vi "Execute.vi"(8 "Error In":errorcluster, 11 "Test Framework.lvclass":refnum<class "Test Framework.lvclass">) -> (0 "Error Out":errorcluster, 3 "Test Framework.lvclass Out":refnum<class "Test Framework.lvclass">)   [LabVIEW 2020, in "Test Framework.lvclass"]
uses:
  Test Framework.lvclass
  Controls/Control references.ctl
  Support VIs/Message Queue/States.ctl
  Controls/Display states.ctl
  Test Framework.lvclass/Test Framework.ctl
  XML Handler/XML Handler.lvclass/XML Handler.ctl
  Instruments/Vector Network Analyzer/Vector Network Analyzer.lvclass
  Path Control/PathControl.lvclass/PathControl.ctl
  Controls/Temperature and voltage modes.ctl
  <vilib>/sound2/lvsound2.llb/Sampling Mode.ctl
  Support VIs/Message Queue/Enqueue Message (Single).vi
  Support VIs/Message Queue/Enqueue Message (Array).vi
  <vilib>/sound2/lvsound2.llb/Sound File Info (path).vi
  <vilib>/sound2/lvsound2.llb/Sound Output Write (DBL).vi
  Devices/Toggle 8/WS1021/WS1021 GUI.vi
  <vilib>/Utility/xml.llb/Write to XML File(string).vi
  Devices/Device.lvclass
  Support VIs/User Event - Stop/User Event - Stop.lvlib
  Support VIs/Message Queue/Message Queue.lvlib
  Path Control/PathControl.lvclass
  XML Handler/XML Handler.lvclass
  Devices/Toggle 8/WS1021/WS1021.lvclass
panel:
  out "Time String":string
  in  "OpenFolder":bool
  in  "Device Information":string[][](array[string])
  in  "File Name":string
  out "Progress Bar":u8(slide) scale=0.0..100.0
  in  "Data Path":path
  in  "Exit Button":bool
  in  "Run Measurements Button":bool
  in  "Configure Measurements Button":bool
  in  "Calibrate Paths Button":bool
  in  "Conf Device Button":bool
  in  "Conf temp and DC Button":bool
  in  "Assign Instr Button":bool
  in  "Test Listbox":i32(listbox) caption="Measurement"
  # "%"
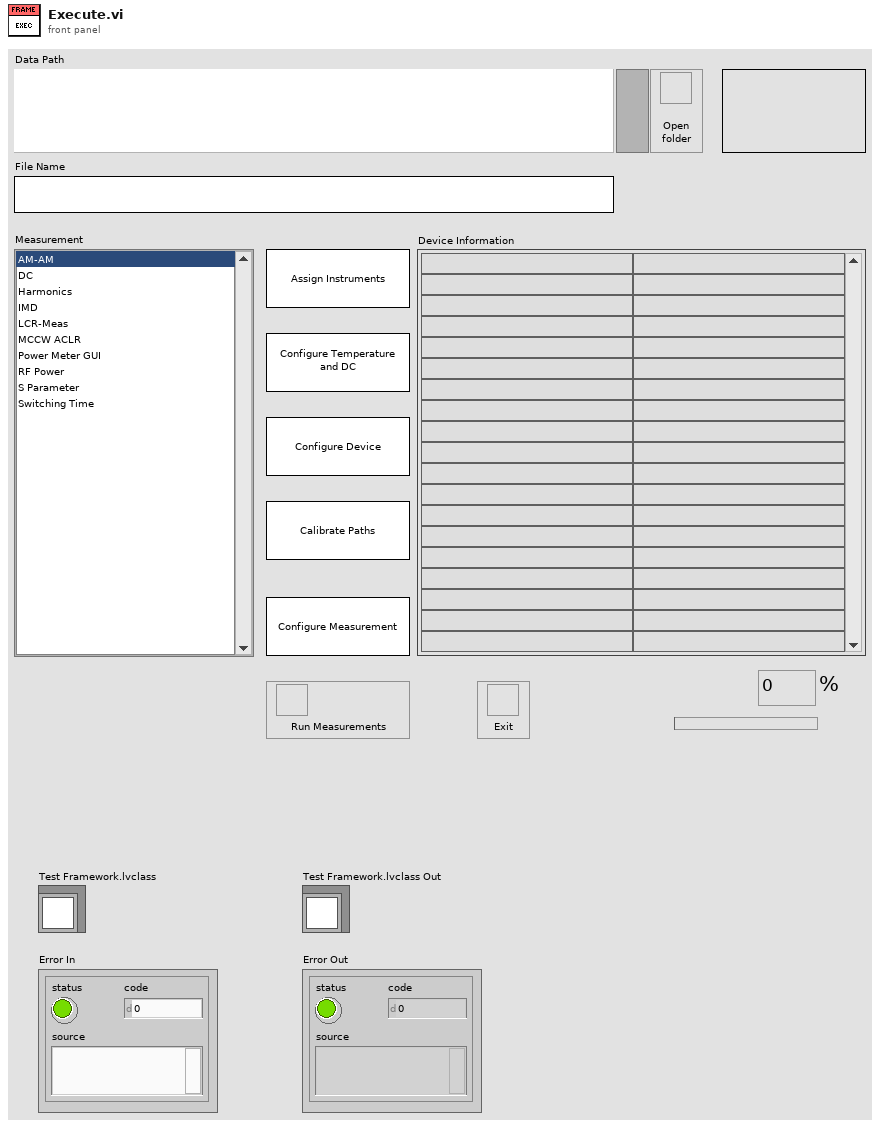
[diagram p1: front panel]
types:
  T1 = enum32{"invalid app kind", "Development System", "Run Time System", "Student Edition", "Embedded LabVIEW", "Evaluation", "Custom"}
  T2 = typedef "Test Framework.lvclass/Control references.ctl" = cluster{"Assign Instr Button Ref":refnum<vi>, "Conf temp/voltage Button Ref":refnum<vi>, "Conf Device Button Ref":refnum<vi>, "Calibrate Path Button Ref":refnum<vi>, "Configure Meas Button Ref":refnum<vi>, "Run Measurements Button Ref":refnum<vi>, "Exit Button Ref":refnum<vi>, "Test Listbox Ref":refnum<vi>, "Data Path Ref":refnum<vi>, "File Name":refnum<vi>, "CtrlWithKeyFocus":refnum<vi>}
  T3 = typedef "Message Queue.lvlib/All Message Queues.ctl" = cluster{"UI":refnum<queue>}
  T4 = enum16{"open", "replace", "create", "open or create", "replace or create", "replace or create with confirmation"}
  T5 = typedef "Test Framework.lvclass/Display states.ctl" = enum16{"Start up", "Measurements Running"}
  T6 = typedef "Message Queue.lvlib/States.ctl" = enum16{"Init", "Update Display", "Assign Instruments", "Configure Evironmental", "Configure Device", "Update device info", "Calibrate Path", "Configure Test", "Init XML", "Init Environmental", "Next Environmental", "Run Tests", "Cancel Tests", "Change Data Path", "Update test list", "Finish test", "Exit", "Error", "Menu Selection"}
  T7 = typedef "Test Framework.lvclass/Temperature and voltage modes.ctl" = cluster{"Temperature mode":enum16{"Automatic", "Manual", "Off"}, "DC-Power mode":enum16{"Automatic", "Manual", "Off"}, "PSU sweep mode":bool, "Turn off after measurement":bool}
  T8 = enum32{"Invalid", "Standard", "Closed", "Hidden", "Minimized", "Maximized"}
  T9 = typedef "Device.lvclass/Device Information Cluster.ctl" = cluster{"Device Info":string[][], "Default Values":T10[], "Fetched info":string[][]}
  T10 = typedef "PIC-Device.lvclass/Register to Write.ctl" = cluster{"Register":u32, "Value":u32, "Dev Address":u32, "Physical Adress":u32}
  T11 = cluster{"Instrument Name":string, "Instrument.lvclass":refnum<class "Instrument.lvclass">, "Reference":bool}[]
  T12 = cluster{"Restart?":bool, "User system setting file":path}
  T13 = typedef "Test Framework.lvclass/Temperature and voltage array.ctl" = cluster{"Temperature [C]":dbl, "Soak time [m]":dbl, "PSUs":cluster{"Enabled":bool, "Source":enum32{"Voltage", "Current"}, "Drive (V/A)":dbl, "Sweep (V/A)":string, "Limit (A/V)":dbl, "PSU alias":string, "PSU info":cluster{"ID":string, "Address":string, "Channel":u8}}[]}[]
  T14 = cluster{"Temperature control array":T13, "Temperature mode":T7}
  T15 = typedef "Sampling Mode.ctl" = i32
  T16 = typedef "Sound Data Format.ctl" = cluster{"sample rate (S/s)":dbl, "number of channels":i32, "bits per sample":i32}
  T17 = typedef "Sound Output Task ID.ctl" = u32
  T18 = enum32{"Bad", "Idle", "Run top level", "Running"}
  T19 = typedef "LVPoint32TypeDef.ctl" = cluster{"Horizontal":i32, "Vertical":i32}
  T20 = cluster{"appended path":path, "appended path":path}
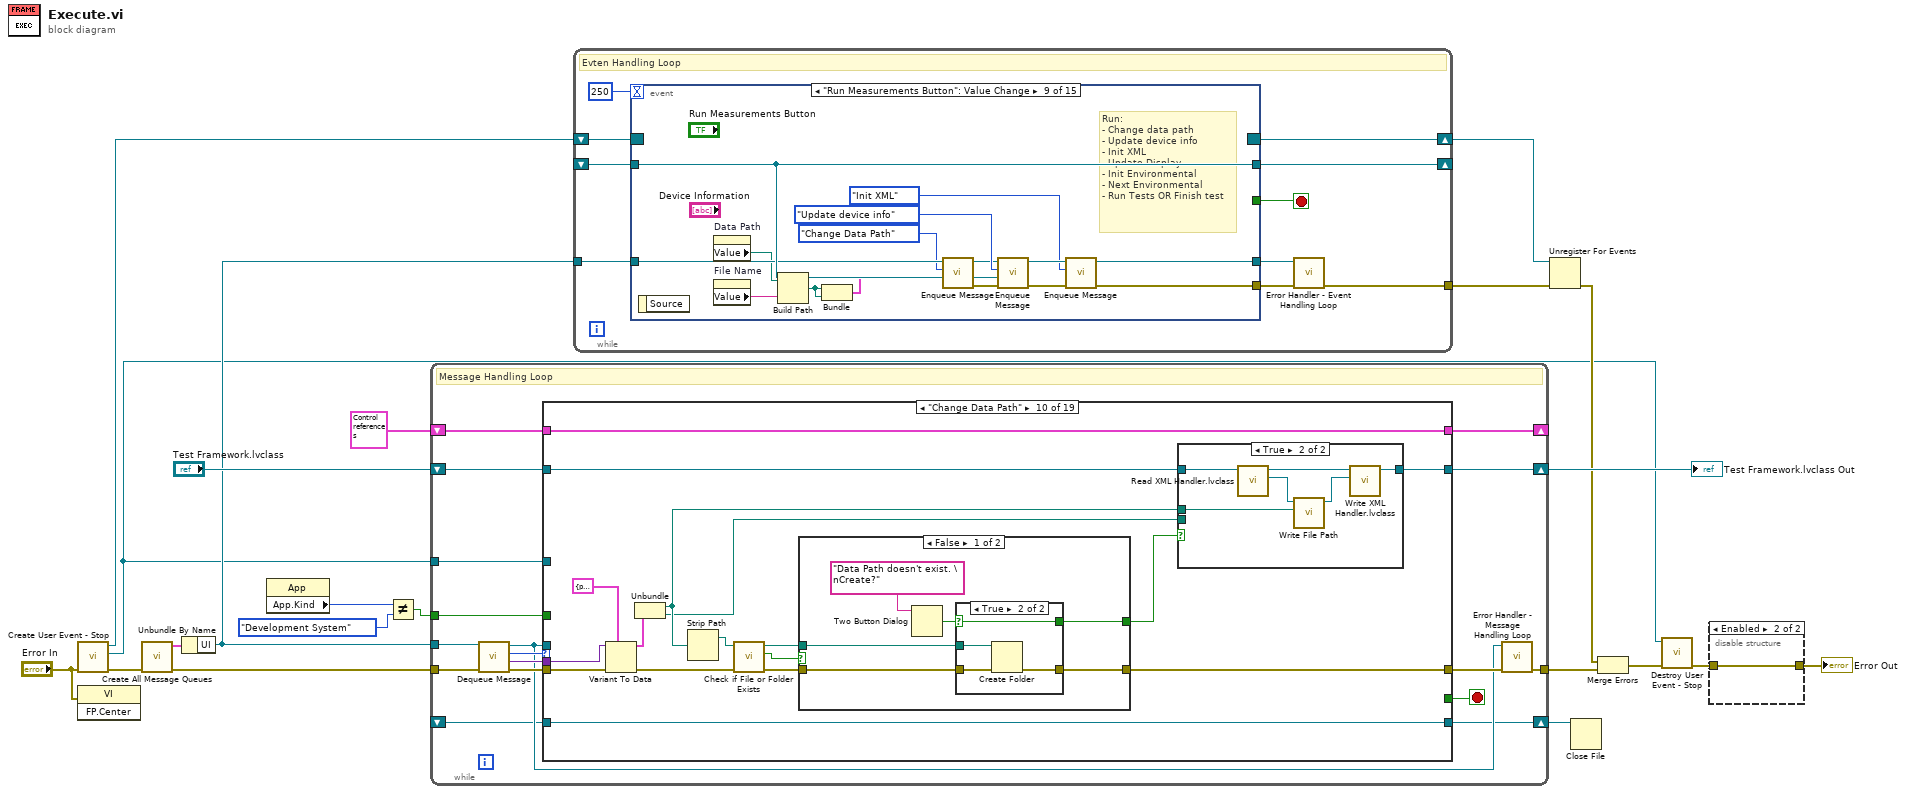
[diagram p0: block diagram]
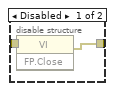
[diagram p2: hidden frame]
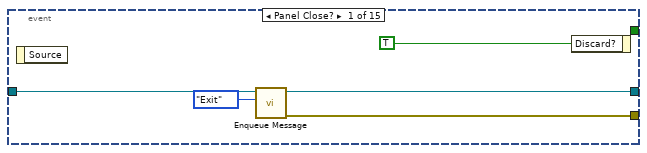
[diagram p3: hidden frame]
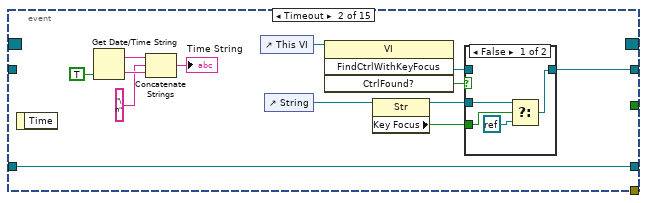
[diagram p4: hidden frame]
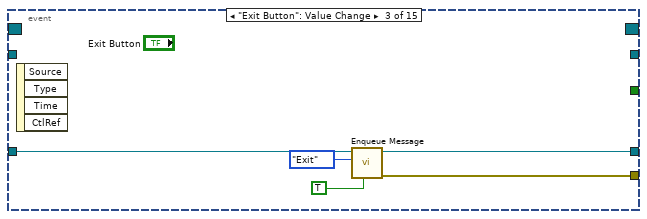
[diagram p6: hidden frame]
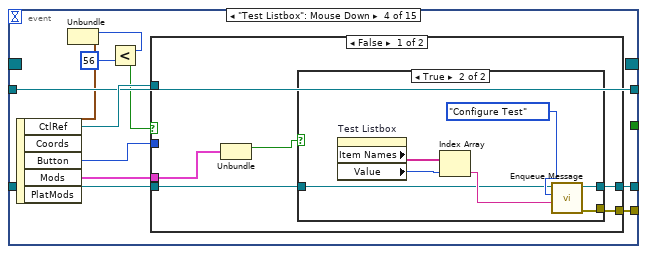
[diagram p7: hidden frame]
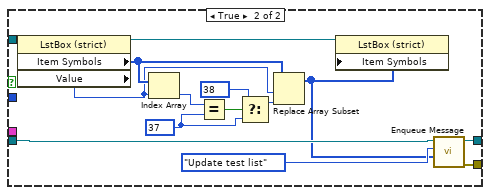
[diagram p9: hidden frame]
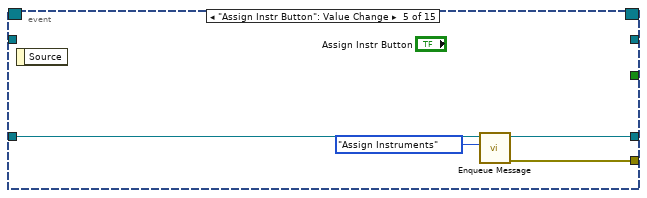
[diagram p10: hidden frame]
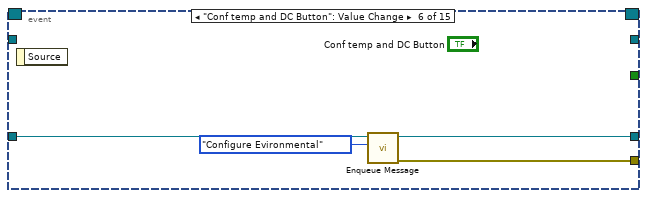
[diagram p11: hidden frame]
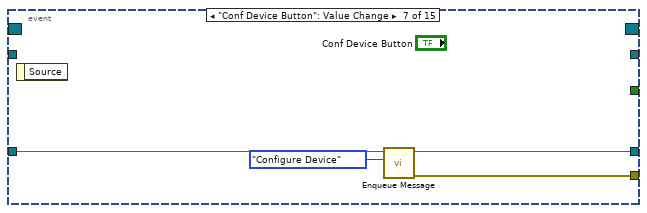
[diagram p12: hidden frame]
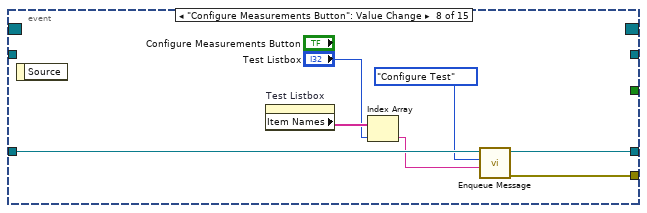
[diagram p13: hidden frame]
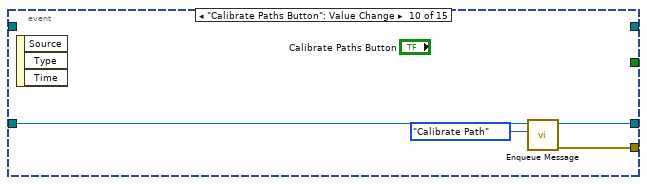
[diagram p14: hidden frame]
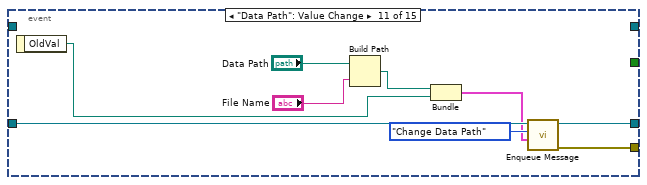
[diagram p15: hidden frame]
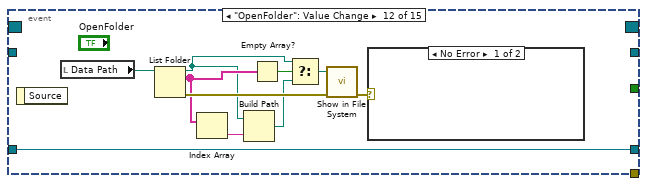
[diagram p16: hidden frame]
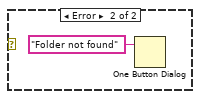
[diagram p17: hidden frame]
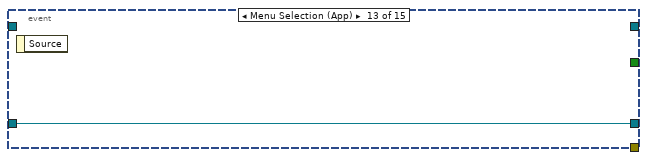
[diagram p18: hidden frame]
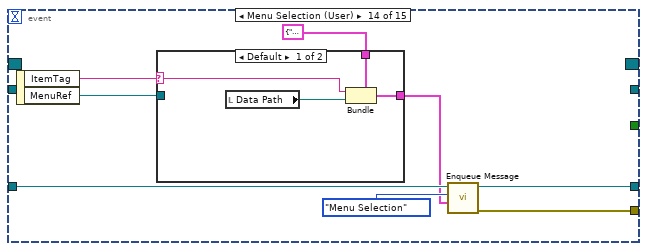
[diagram p19: hidden frame]
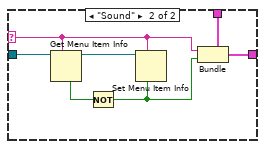
[diagram p20: hidden frame]
diagram:
  n1 = call "Create User Event - Stop.vi"("error in (no error)"="Error In") -> ("error out"=w21:errorcluster, "User Event - Stop"=w10:refnum<user-event>, "Stop Event Registration Refnum"=w15:refnum<event-registration>)  [unwired: 8 in]
  n2 = invoke class="VI" method="FP.Center"(error in="Error In") -> ()  [unwired: 2 in, 3 out]
  n3 = call "Create All Message Queues.vi"("error in (no error)"=w21) -> ("error out"=w20:errorcluster, "Message Queues out"=w19:T3)  [unwired: 9 in]
  n4 = Unbundle By Name(w19) -> ("UI"=w16:refnum<queue>)
  n5 = property class="App"() -> ("App.Kind"=w2:T1)  [unwired: 2 in, 2 out]
  n6 = Not Equal?(x=w2, y=T1."Development System" ("Application:Kind")) -> (x != y?=w1:bool)
  n7 = while {
    tunnel: w16 -> [w37]
    shift-right: [w32] -> w17
    shift-left: "Test Framework.lvclass" -> [w33]
    tunnel: w20 -> [w38]
    tunnel: w10 -> [w31]
    tunnel: [w27] -> w11
    shift-right: [w25] -> _
    shift-left: T2 {"Assign Instr Button Ref"=refnum, "Conf temp/voltage Button Ref"=refnum, "Conf Device Button Ref"=refnum, "Calibrate Path Button Ref"=refnum, "Configure Meas Button Ref"=refnum, "Run Measurements Button Ref"=refnum, "Exit Button Ref"=refnum, "Test Listbox Ref"=refnum, "Data Path Ref"=refnum, "File Name"=refnum, "CtrlWithKeyFocus"=refnum} ("Cluster") -> [w26]
    shift-right: [w23] -> w4
    shift-left: _ -> [w24]
    tunnel: w1 -> [w22]
    stop <- w30 stop-if-true
    # "Message Handling Loop"
    n8 = call "Dequeue Message.vi"("error in (no error)"=w38, "Message Queue"=w37) -> ("error out"=w35:errorcluster, "Message Data"=w34:variant, "Message"=w36:T6, "dup Message Queue"=w28:refnum<queue>)  [unwired: 6 in]
    n9 = case shown="\"Change Data Path\"" w36 {
      tunnel: w28 -> [w66 _ _ _ _ _ _ w213 _ _ w287 w297 _ w326 w363 _ w410 w434 _]
      tunnel: w35 -> [w45 w91 w99 w106 w140 w161 w192 w220 w239 w256 w292 w305 w315 w331 w365 w391 w414 w419 w470]
      tunnel: w34 -> [_ w88 _ _ w139 _ w191 _ _ w255 _ w304 _ w324 _ w389 _ _ w469]
      tunnel: w33 -> [w84 w93 w97 w107 w149 w167 w195 w211 w238 w254 w283 w306 w314 w330 w361 w395 w413 w417 w461]
      tunnel: [w47 w93 w96 w102 w150 w168 w194 w222 w238 w253 w284 w306 w310 w329 w364 w386 w412 w421 w460] -> w32
      tunnel: [w67 w92 w98 w105 w141 w171 w193 w215 w239 w240 w288 w295 w311 w325 w362 w390 w409 w428 w466] -> w29
      tunnel: w31 -> [_ _ _ _ _ _ _ _ _ _ w291 _ _ _ _ _ _ _ w458]
      tunnel: [_ _ _ _ _ _ _ _ _ _ TRUE _ _ _ _ _ _ _ w457] -> w30
      tunnel: w26 -> [w78 w85 w95 w108 w136 w160 w187 w221 w237 w252 w286 w300 w309 w328 w366 w396 w415 w423 w471]
      tunnel: [w77 w85 w95 w108 w135 w160 w187 w221 w237 w252 w286 w300 w309 w328 w366 w396 w415 w423 w471] -> w25
      tunnel: w24 -> [_ w86 w94 w100 w142 w159 w186 w201 w236 w251 w285 w294 w307 w322 w341 w385 w401 w426 w468]
      tunnel: [w53 w86 w94 w100 w142 w159 w186 w201 w236 w251 w285 w293 w307 w322 w341 w385 w401 w426 w468] -> w23
      tunnel: w22 -> [_ _ _ _ _ _ _ _ _ _ _ _ _ _ _ _ _ _ w459]
      frame "Init" {
        n10 = call "Read Test Listbox.vi"("Test Framework in"=w84) -> ("Value"=w81:i32, "Symbols"=w82:i32[], "Measurement Names"=w83:string[], "Test Framework out"=w80:refnum<class "Test Framework.lvclass">)  [unwired: 7 in]
        n11 = call "Get AppData Directory.vi"("Error In"=w45) -> ("Error Out"=w44:errorcluster, "Folder path"=w43:path)  [unwired: 8 in, 1 out]
        n12 = property on="Test Listbox" class="LstBox (strict)"("Item Names"=w83, "Item Symbols"=w82, "Value"=w81) -> ()  [unwired: 2 in, 2 out]
        n13 = call "Read XML Handler.lvclass.vi"("Test Framework in"=w80) -> ("XML Handler.lvclass"=w79:refnum<class "XML Handler.lvclass">, "Test Framework out"=w60:refnum<class "Test Framework.lvclass">)  [unwired: 9 in]
        n14 = call "Read File Path.vi"("XML Handler in"=w79) -> ("File Path"=w62:path)  [unwired: 9 in, 1 out]
        n15 = call-dynamic "Read Current Device.vi"("Test Framework in"=w60) -> ("Current Device.lvclass"=w61:refnum<class "Device.lvclass">, "Test Framework out"=w48:refnum<class "Test Framework.lvclass">)  [unwired: 9 in]
        n16 = Strip Path(path=w62) -> (stripped path=w63:path)  [unwired: 1 out]
        n17 = call <vilib>:"Get File Extension.vi"("file"=w62) -> ("filename without extension"=w41:string)  [unwired: 6 in, 4 out]
        n18 = Build Path(base path=w43, name or relative path="Error Log.txt") -> (appended path=w56:path)
        n19 = call-dynamic "Read Device Information.vi"("Device in"=w61) -> ("Device Info"=w59:T9[])  [unwired: 8 in, 2 out]
        n20 = Empty String/Path?(string/path=w41) -> (empty?=w42:bool)
        n21 = property on="Data Path" class="Path"("Value"=w63) -> ()  [unwired: 2 in, 2 out]
        n22 = Open/Create/Replace File(file path (use dialog)=w56, error in=w44, operation (0:open)=T4."open or create") -> (refnum out=w53:refnum<file>, error out=w52:errorcluster)  [unwired: 3 in, 1 out]
        n23 = Select(t="results", s=w42, f=w41) -> (s? t:f=w39:string)
        n24 = Index Array(array=w59) -> (element=w58:T9)  [unwired: 1 in]
        n25 = call-dynamic "Read Play sound when done.vi"("Test Framework in"=w48) -> ("Play sound when done"=w46:bool, "Test Framework out"=w47:refnum<class "Test Framework.lvclass">)  [unwired: 9 in]
        n26 = property on="File Name" class="Str"("Value"=w39) -> ()  [unwired: 2 in, 2 out]
        n27 = Unbundle By Name(w58) -> ("Device Info"=w57:string[][])
        n28 = control-ref of="Assign Instr Button"() -> (w76:refnum<vi>)
        n29 = control-ref of="Conf temp and DC Button"() -> (w75:refnum<vi>)
        n30 = control-ref of="Conf Device Button"() -> (w74:refnum<vi>)
        n31 = control-ref of="Calibrate Paths Button"() -> (w73:refnum<vi>)
        n32 = control-ref of="Configure Measurements Button"() -> (w72:refnum<vi>)
        n33 = control-ref of="Run Measurements Button"() -> (w71:refnum<vi>)
        n34 = control-ref of="Exit Button"() -> (w70:refnum<vi>)
        n35 = control-ref of="Test Listbox"() -> (w69:refnum<vi>)
        n36 = control-ref of="File Name"() -> (w51:refnum<vi>)
        n37 = control-ref of="Data Path"() -> (w68:refnum<vi>)
        n38 = local write "Device Information"(w57) -> ()
        n39 = Current VI's Menubar() -> (w50:refnum<k9>)
        n40 = Set Menu Item Info(6:w46, 7:"Sound" ("item tag"), 11:w50) -> ()  [unwired: 4 in, 2 out]
        n41 = Bundle By Name(cluster=w78, "Assign Instr Button Ref"=w76, "Conf temp/voltage Button Ref"=w75, "Conf Device Button Ref"=w74, "Calibrate Path Button Ref"=w73, "Configure Meas Button Ref"=w72, "Run Measurements Button Ref"=w71, "Exit Button Ref"=w70, "Test Listbox Ref"=w69, "Data Path Ref"=w68, "File Name"=w51) -> (w77:T2)
        n42 = call-poly "Enqueue Message.vi"("error in (no error)"=w52, "Message Data"=Display_states."Start up" ("type"), "Message"=States."Update Display", "Message Queue"=w66) -> ("error out"=w67:errorcluster)  [unwired: 6 in, 1 out]
      }
      frame "Update Display" {
        n43 = Variant To Data(error in=w91, type=Display_states."Start up", Variant=w88) -> (data=w90:T5, error out=w89:errorcluster)
        n44 = call "Update display.vi"("Error In"=w89, "Display states"=w90, "Cluster"=w85) -> ("Error Out"=w92:errorcluster)  [unwired: 8 in]
      }
      frame "Configure Evironmental" {
        n45 = call "Configure Environment.vi"("error in (no error)"=w99, "Test Framework in"=w97) -> ("error out"=w98:errorcluster, "Test Framework out"=w96:refnum<class "Test Framework.lvclass">)  [unwired: 8 in]
      }
      frame "Configure Device" {
        n46 = local read "Device Information"() -> (w101:string[][])
        n47 = call "Select Device.vi"("Error In"=w106, "Test Framework.lvclass"=w107) -> ("Error Out"=w105:errorcluster, "Test Framework out"=w103:refnum<class "Test Framework.lvclass">)  [unwired: 8 in]
        n48 = call-dynamic "Read Current Device.vi"("Test Framework in"=w103) -> ("Current Device.lvclass"=w104:refnum<class "Device.lvclass">, "Test Framework out"=w102:refnum<class "Test Framework.lvclass">)  [unwired: 9 in]
        n49 = disable-structure shown="Disabled" {
          disable-tunnel: w104 -> [w114 _]
          disable-tunnel: w101 -> [w112 _]
          frame Disabled {
            n50 = call-dynamic "Read Device Information.vi"("Device in"=w114) -> ("Device Info"=w113:T9[])  [unwired: 8 in, 2 out]
            n51 = for {
              tunnel: w113 -> [w121] mode=indexing
              tunnel: [w117] -> w110 mode=indexing if=w116
              shift-right: [w115] -> w111
              shift-left: w112 -> [w120]
              n52 = Index Array(array=w120) -> (element #1=w119:string[], element #2=w118:string[])  [unwired: 4 in]
              n53 = for {
                tunnel: w119 -> [w132] mode=indexing
                tunnel: w118 -> [w126] mode=indexing
                tunnel: [w131] -> w115 mode=indexing
                tunnel: [w122] -> w116
                tunnel: w121 -> [w128]
                tunnel: [w123] -> w117
                stop <- w122 continue-if-true
                n54 = Unbundle By Name(w128) -> ("Fetched info"=w130:string[][])
                n55 = Index Array(array=w130) -> (element=w129:string[])  [unwired: 2 in]
                n56 = Unbundle(w129) -> (w125, w124)
                n57 = Not Equal?(x=w132, y=w125) -> (x != y?=w122:bool)
                n58 = Select(t=w126, s=w122, f=w124) -> (s? t:f=w127:string)
                n59 = Build Array(w132, w127) -> (w131:string[])
                n60 = Build Array(w125, w124) -> (w123:void[])
              }
            }
            n61 = Insert Into Array(array=w111, new element=w110) -> (w109:string[][])  [unwired: 2 in]
            n62 = local write "Device Information"(w109) -> ()
          }
          frame Enabled {
          }
        }
      }
      frame "Update device info" {
        n63 = Variant To Data(error in=w140, type=refnum<vi> refnum ("CtrlWithKeyFocus"), Variant=w139) -> (data=w137:refnum<vi>, error out=w141:errorcluster)
        n64 = call-dynamic "Read Current Device.vi"("Test Framework in"=w149) -> ("Current Device.lvclass"=w145:refnum<class "Device.lvclass">, "Test Framework out"=w144:refnum<class "Test Framework.lvclass">)  [unwired: 9 in]
        n65 = Bundle By Name(cluster=w136, "CtrlWithKeyFocus"=w137) -> (w135:T2)
        n66 = local read "Device Information"() -> (w134:string[][])
        n67 = for {
          tunnel: w134 -> [w153] mode=indexing
          tunnel: [w153] -> w133 mode=indexing if=w151
          n68 = Index Array(array=w153, index=1) -> (element=w154:string)
          n69 = Empty String/Path?(string/path=w154) -> (empty?=w152:bool)
          n70 = Not(x=w152) -> (.not. x?=w151:bool)
        }
        n71 = call-dynamic "Read Device Information.vi"("Device in"=w145) -> ("Device Info"=w148:T9[], "Device out"=w146:refnum<class "Device.lvclass">)  [unwired: 8 in, 1 out]
        n72 = for {
          tunnel: w148 -> [w158] mode=indexing
          tunnel: [w157] -> w147 mode=indexing
          tunnel: w133 -> [w156]
          n73 = Bundle By Name(cluster=w158, "Device Info"=w156) -> (w157:T9)
        }
        n74 = call-dynamic "Write Device Information.vi"("Device Info"=w147, "Device in"=w146) -> ("Device out"=w143:refnum<class "Device.lvclass">)  [unwired: 8 in, 1 out]
        n75 = call-dynamic "Write Current Device.vi"("Current Device.lvclass"=w143, "Test Framework in"=w144) -> ("Test Framework out"=w150:refnum<class "Test Framework.lvclass">)  [unwired: 9 in]
      }
      frame "Calibrate Path" {
        n76 = call "Read PathControl.lvclass.vi"("Test Framework in"=w167) -> ("PathControl.lvclass"=w163:refnum<class "PathControl.lvclass">, "Test Framework out"=w170:refnum<class "Test Framework.lvclass">)  [unwired: 9 in]
        n77 = call "Read Instrumentes to Use.vi"("Test Framework in"=w167) -> ("Instrumentes to Use"=w166:T11)  [unwired: 9 in, 1 out]
        n78 = call "Find Instrument.vi"("Instrument Name"="Vector Network Analyzer", "Instrumentes to Use"=w166) -> ("Instrument Found?"=w164:bool, "Instrument.lvclass"=w162:refnum<class "Instrument.lvclass">)  [unwired: 8 in]
        n79 = case shown="True" w164 {
          tunnel: [w180 w185] -> w171
          tunnel: [w179 w184] -> w169
          tunnel: w163 -> [w177 w181]
          tunnel: w162 -> [w176 _]
          tunnel: w161 -> [w173 w183]
          frame True {
            n80 = To More Specific Class(target class=refnum<class "Vector Network Analyzer.lvclass"> refnum ("Vector Network Analyzer.lvclass"), reference=w176) -> (specific class reference=w174:refnum<class "Vector Network Analyzer.lvclass">)  [unwired: 1 in, 1 out]
            n81 = call "Write Vector Network Analyzer.lvclass.vi"("Vector Network Analyzer.lvclass"=w174, "PathControl in"=w177) -> ("PathControl out"=w178:refnum<class "PathControl.lvclass">)  [unwired: 9 in]
            n82 = call "Calibrate Path User Interface.vi"("error in (no error)"=w173, "VNA present"=TRUE ("VNA pressent"), "PathControl in"=w178) -> ("error out"=w180:errorcluster, "PathControl out"=w179:refnum<class "PathControl.lvclass">)  [unwired: 7 in]
          }
          frame False {
            n83 = call "Calibrate Path User Interface.vi"("error in (no error)"=w183, "VNA present"=FALSE ("VNA pressent"), "PathControl in"=w181) -> ("error out"=w185:errorcluster, "PathControl out"=w184:refnum<class "PathControl.lvclass">)  [unwired: 7 in]
          }
        }
        n84 = call "Write PathControl.lvclass.vi"("PathControl.lvclass"=w169, "Test Framework in"=w170) -> ("Test Framework out"=w168:refnum<class "Test Framework.lvclass">)  [unwired: 9 in]
      }
      frame "Configure Test" {
        n85 = Variant To Data(error in=w192, type="", Variant=w191) -> (data=w188:string, error out=w189:errorcluster)
        n86 = call "Configure Measurement.vi"("error in (no error)"=w189, "Measurement Name"=w188, "Test Framework in"=w195) -> ("error out"=w193:errorcluster, "Test Framework out"=w194:refnum<class "Test Framework.lvclass">)  [unwired: 7 in]
      }
      frame "Run Tests" {
        n87 = call-dynamic "Read Current Device.vi"("Test Framework in"=w211) -> ("Current Device.lvclass"=w209:refnum<class "Device.lvclass">, "Test Framework out"=w212:refnum<class "Test Framework.lvclass">)  [unwired: 9 in]
        n88 = local read "Device Information"() -> (w205:string[][])
        n89 = Unbundle By Name(w221) -> ("Test Listbox Ref"=w219:refnum<vi>)
        n90 = property class="Device.lvclass"(reference=w209) -> (reference out=w203:refnum<class "Device.lvclass">, "Accessors:Device Info"=w208:T9[])  [unwired: 1 in, 1 out]
        n91 = property class="LstBox (strict)"(reference=w219) -> ("Item Names"=w218:string[], "Item Symbols"=w217:i32[])  [unwired: 1 in, 2 out]
        n92 = Index Array(array=w208) -> (element=w206:T9)  [unwired: 1 in]
        n93 = Bundle By Name(cluster=w206, "Device Info"=w205) -> (w204:T9)
        n94 = Build Array(w204) -> (w207:T9[])
        n95 = for {
          tunnel: w218 -> [w227] mode=indexing
          tunnel: w217 -> [w229] mode=indexing
          tunnel: [w227] -> w216 mode=indexing if=w226
          n96 = Equal?(x=w229, y=38) -> (x = y?=w226:bool)
        }
        n97 = property class="Device.lvclass"(reference=w203, "Accessors:Device Info"=w207) -> (reference out=w202:refnum<class "Device.lvclass">)  [unwired: 1 in, 1 out]
        n98 = call-dynamic "Write Current Device.vi"("Current Device.lvclass"=w202, "Test Framework in"=w212) -> ("Test Framework out"=w210:refnum<class "Test Framework.lvclass">)  [unwired: 9 in]
        n99 = for {
          shift-right: [w231] -> w214
          shift-left: w220 -> [w233]
          tunnel: w216 -> [w232] mode=indexing
          shift-right: [w234] -> w222
          shift-left: w210 -> [w235]
          tunnel: [w230] -> w200
          stop <- w230 stop-if-true
          n100 = call "Run Test.vi"("error in (no error)"=w233, "Measurement Name"=w232, "Test Framework in"=w235) -> ("error out"=w231:errorcluster, "Canceled"=w230:bool, "Test Framework out"=w234:refnum<class "Test Framework.lvclass">)  [unwired: 6 in]
        }
        n101 = case shown="True" w200 {
          tunnel: [FALSE ("T button?") w224] -> w199
          frame False {
          }
          frame True {
            n102 = Two Button Dialog(message="Stop execution of the measurement queue?") -> (T button?=w224:bool)  [unwired: 2 in]
          }
        }
        n103 = Select(t=States."Finish test" ("Message"), s=w199, f=States."Next Environmental" ("Message")) -> (s? t:f=w198:T6)
        n104 = call-poly "Enqueue Message.vi"("error in (no error)"=w214, "Message"=w198, "Message Queue"=w213) -> ("error out"=w215:errorcluster)  [unwired: 7 in, 1 out]
      }
      frame "Cancel Tests" {
      }
      frame "Change Data Path" {
        n105 = Variant To Data(error in=w256, type=cluster{"appended path":path, "OldVal":path} {"appended path"=path "", "OldVal"=path ""} ("cluster"), Variant=w255) -> (data=w245:cluster{"appended path":path, "OldVal":path}, error out=w249:errorcluster)
        n106 = Unbundle(w245) -> ("appended path"=w244:path, "OldVal"=w242:path)
        n107 = Strip Path(path=w244) -> (stripped path=w250:path)  [unwired: 1 out]
        n108 = call <vilib>:"Check if File or Folder Exists.vi"("error in (no error)"=w249, "path"=w250) -> ("error out"=w247:errorcluster, "file or folder exists?"=w248:bool, "dup path"=w243:path)  [unwired: 7 in]
        n109 = case shown="False" w248 {
          selector: w248 -> [_ w278]
          tunnel: w247 -> [w267 w277]
          tunnel: w243 -> [w268 _]
          tunnel: [w266 w277] -> w240
          tunnel: [w265 w278] -> w241
          frame False {
            n110 = Two Button Dialog(message="Data Path doesn't exist. \nCreate?") -> (T button?=w269:bool)  [unwired: 2 in]
            n111 = case shown="True" w269 {
              selector: w269 -> [w271 w273]
              tunnel: w268 -> [_ w276]
              tunnel: w267 -> [w272 w275]
              tunnel: [w272 w274] -> w266
              tunnel: [w271 w273] -> w265
              frame False {
              }
              frame True {
                n112 = Create Folder(path (use dialog)=w276, error in=w275) -> (error out=w274:errorcluster)  [unwired: 1 in, 2 out]
              }
            }
          }
          frame True {
          }
        }
        n113 = case shown="True" w241 {
          tunnel: w254 -> [w258 w264]
          tunnel: [w258 w260] -> w253
          tunnel: w244 -> [_ w259]
          tunnel: w242 -> [w257 _]
          frame False {
            n114 = property on="Data Path" class="Path"("Val(Sgnl)"=w257) -> ()  [unwired: 2 in, 2 out]
          }
          frame True {
            n115 = call "Read XML Handler.lvclass.vi"("Test Framework in"=w264) -> ("XML Handler.lvclass"=w262:refnum<class "XML Handler.lvclass">, "Test Framework out"=w263:refnum<class "Test Framework.lvclass">)  [unwired: 9 in]
            n116 = call "Write File Path.vi"("File Path"=w259, "XML Handler in"=w262) -> ("XML Handler out"=w261:refnum<class "XML Handler.lvclass">)  [unwired: 9 in]
            n117 = call "Write XML Handler.lvclass.vi"("XML Handler.lvclass"=w261, "Test Framework in"=w263) -> ("Test Framework out"=w260:refnum<class "Test Framework.lvclass">)  [unwired: 9 in]
          }
        }
      }
      frame "Exit" {
        n118 = call-dynamic "Read User system setting file.vi"("Test Framework in"=w283) -> ("User system setting file"=w281:T12, "Test Framework out"=w282:refnum<class "Test Framework.lvclass">)  [unwired: 9 in]
        n119 = Bundle By Name(cluster=w281, "Restart?"=FALSE) -> (w280:T12)
        n120 = call-dynamic "Write User system setting file.vi"("User system setting file"=w280, "Test Framework in"=w282) -> ("Test Framework out"=w284:refnum<class "Test Framework.lvclass">)  [unwired: 9 in]
        n121 = call "Fire User Event - Stop.vi"("error in (no error)"=w292, "User Event - Stop"=w291) -> ("error out"=w289:errorcluster)  [unwired: 9 in]
        n122 = Release Queue(queue=w287, error in (no error)=w289) -> (error out=w288:errorcluster)  [unwired: 1 in, 2 out]
      }
      frame "Error", Default {
        n123 = Variant To Data(error in=w305, type=errorcluster {"status"=FALSE, "code"=0, "source"=""} ("error constant"), Variant=w304) -> (data=w302:errorcluster)  [unwired: 1 out]
        n124 = call "Error Handler.vi"("Error In"=w302, "refnum in"=w294) -> ("Error Out"=w301:errorcluster, "refnum out"=w293:refnum<file>)  [unwired: 8 in]
        n125 = call <vilib>:"Clear Errors.vi"("error in (no error)"=w301) -> ("error out"=w296:errorcluster)  [unwired: 5 in, 1 out]
        n126 = call-poly "Enqueue Message.vi"("error in (no error)"=w296, "Message Data"=Display_states."Start up" ("type"), "Message"=States."Update Display", "Message Queue"=w297) -> ("error out"=w295:errorcluster)  [unwired: 6 in, 1 out]
      }
      frame "Assign Instruments" {
        n127 = call "Assign Instruments.vi"("error in (no error)"=w315, "Test Framework in"=w314) -> ("error out"=w312:errorcluster, "Canceled"=w308:bool, "Test Framework out"=w313:refnum<class "Test Framework.lvclass">)  [unwired: 7 in]
        n128 = case shown="False" w308 {
          tunnel: w313 -> [w319 w320]
          tunnel: w312 -> [w318 w321]
          tunnel: [w317 w321] -> w311
          tunnel: [w316 w320] -> w310
          frame False {
            n129 = call "Found to Used instruments.vi"("error in (no error)"=w318, "Test Framework in"=w319) -> ("error out"=w317:errorcluster, "Test Framework out"=w316:refnum<class "Test Framework.lvclass">)  [unwired: 8 in]
          }
          frame True {
          }
        }
      }
      frame "Init Environmental" {
        n130 = local write "Progress Bar"(u8 0 ("Horizontal Progress Bar")) -> ()
        n131 = call "Init Environment.vi"("error in (no error)"=w331, "Test Framework in"=w330) -> ("error out"=w327:errorcluster, "Test Framework out"=w329:refnum<class "Test Framework.lvclass">)  [unwired: 8 in]
        n132 = case shown="No Error" w327 {
          selector: w327 -> [w336 w340]
          tunnel: w326 -> [w335 w337]
          tunnel: [w334 w340] -> w325
          tunnel: w324 -> [w332 _]
          frame No Error {
            n133 = call-poly "Enqueue Message.vi"("error in (no error)"=w336, "Message Data"=w332, "Message"=States."Next Environmental", "Message Queue"=w335) -> ("error out"=w334:errorcluster)  [unwired: 6 in, 1 out]
          }
          frame Error {
            n134 = call-poly "Enqueue Message.vi"("Message Data"=Display_states."Start up" ("type"), "Message"=States."Update Display", "Message Queue"=w337) -> ()  [unwired: 7 in, 2 out]
          }
        }
      }
      frame "Next Environmental" {
        n135 = call-dynamic "Read Temperature control.vi"("Test Framework in"=w361) -> ("Temperature control"=w358:T14, "Test Framework out"=w360:refnum<class "Test Framework.lvclass">)  [unwired: 9 in]
        n136 = call "Read Temperature index.vi"("Test Framework in"=w361) -> ("Environmental index"=w346:i32)  [unwired: 9 in, 1 out]
        n137 = Unbundle(w358) -> ("Temperature control array"=w359:T13, "Temperature mode"=w355:T7)
        n138 = Unbundle(w355) -> ("Temperature mode"=w353:enum16{"Automatic", "Manual", "Off"}, "DC-Power mode"=w351:enum16{"Automatic", "Manual", "Off"})  [unwired: 2 out]
        n139 = Array Size(array=w359) -> (size(s)=w345:i32)
        n140 = Unbundle(T7 {"Temperature mode"=enum."Off", "DC-Power mode"=enum."Off", "PSU sweep mode"=FALSE, "Turn off after measurement"=FALSE} ("Temperature mode")) -> ("Temperature mode"=w352:enum16{"Automatic", "Manual", "Off"}, "DC-Power mode"=w350:enum16{"Automatic", "Manual", "Off"})  [unwired: 2 out]
        n141 = Divide(x=w346, y=w345) -> (x/y=w344:dbl)
        n142 = Not Equal?(x=w353, y=w352) -> (x != y?=w349:bool)
        n143 = Multiply(x=w344, y=100.0) -> (x*y=→"Progress Bar":dbl)
        n144 = Not Equal?(x=w351, y=w350) -> (x != y?=w348:bool)
        n145 = Or(x=w349, y=w348) -> (x .or. y?=w347:bool)
        n146 = Greater Than 0?(x=w346) -> (x > 0?=w357:bool)
        n147 = Equal?(x=w345, y=w346) -> (x = y?=w354:bool)
        n148 = case shown="False" w354 {
          tunnel: w365 -> [w379 w380]
          tunnel: [w378 w381] -> w364
          tunnel: w363 -> [w376 w383]
          tunnel: [w374 w384] -> w362
          tunnel: w360 -> [w371 w381]
          tunnel: w347 -> [w370 _]
          tunnel: w357 -> [w367 _]
          frame False {
            n149 = call "Next Environment.vi"("error in (no error)"=w379, "Test Framework in"=w371) -> ("error out"=w377:errorcluster, "User canceled"=w369:bool, "Test Framework out"=w378:refnum<class "Test Framework.lvclass">)  [unwired: 7 in]
            n150 = Select(t=w369, s=w370, f=w367) -> (s? t:f=w368:bool)
            n151 = Select(t=States."Finish test" ("Message"), s=w368, f=States."Run Tests" ("t")) -> (s? t:f=w375:T6)
            n152 = call-poly "Enqueue Message.vi"("error in (no error)"=w377, "Message"=w375, "Message Queue"=w376) -> ("error out"=w374:errorcluster)  [unwired: 7 in, 1 out]
          }
          frame True {
            n153 = call-poly "Enqueue Message.vi"("error in (no error)"=w380, "Message"=States."Finish test", "Message Queue"=w383) -> ("error out"=w384:errorcluster)  [unwired: 7 in, 1 out]
          }
        }
      }
      frame "Update test list" {
        n154 = Variant To Data(error in=w391, type=i32[] [] ("Item Symbols"), Variant=w389) -> (data=w387:i32[], error out=w390:errorcluster)
        n155 = call "Read Test Listbox.vi"("Test Framework in"=w395) -> ("Value"=w392:i32, "Measurement Names"=w393:string[], "Test Framework out"=w394:refnum<class "Test Framework.lvclass">)  [unwired: 7 in, 1 out]
        n156 = call "Write Test Listbox.vi"("Value"=w392, "Symbols"=w387, "Measurement Names"=w393, "Test Framework in"=w394) -> ("Test Framework out"=w386:refnum<class "Test Framework.lvclass">)  [unwired: 7 in]
      }
      frame "Init XML" {
        w408 = T6[] [enum."Update Display", enum."Init Environmental"] items=["Init", "Update Display", "Assign Instruments", "Configure Evironmental", "Configure Device", "Update device info", "Calibrate Path", "Configure Test", "Init XML", "Init Environmental", "Next Environmental", "Run Tests", "Cancel Tests", "Change Data Path", "Update test list", "Finish test", "Exit", "Error", "Menu Selection"]
        n157 = property on="File Name" class="Str"() -> ("Value"=w398:string)  [unwired: 2 in, 2 out]
        n158 = Empty String/Path?(string/path=w398) -> (empty?=w400:bool)
        n159 = Select(t="results", s=w400, f=w398) -> (s? t:f=w397:string)
        n160 = property on="Data Path" class="Path"() -> ("Value"=w403:path)  [unwired: 2 in, 2 out]
        n161 = property on="File Name" class="Str"("Val(Sgnl)"=w397) -> ()  [unwired: 2 in, 2 out]
        n162 = Build Path(base path=w403, name or relative path=w397) -> (appended path=w402:path)
        n163 = call "Init XML handler.vi"("error in (no error)"=w414, "Output File Folder"=w402, "Test Framework in"=w413) -> ("error out"=w411:errorcluster, "Test Framework out"=w412:refnum<class "Test Framework.lvclass">)  [unwired: 7 in]
        n164 = To Variant(anything=Display_states."Measurements Running" ("type")) -> (Variant=w406:variant)
        n165 = Build Array(w406, variant ("Message Data")) -> (w404:variant[])
        n166 = call-poly "Enqueue Message.vi"("error in (no error)"=w411, "Message Data Array"=w404, "Message Array"=w408, "Message Queue"=w410) -> ("error out"=w409:errorcluster)  [unwired: 6 in, 1 out]
      }
      frame "Finish test" {
        n167 = call "Finish Environment.vi"("error in (no error)"=w419, "Test Framework in"=w417) -> ("error out"=w418:errorcluster, "Test Framework out"=w416:refnum<class "Test Framework.lvclass">)  [unwired: 8 in]
        n168 = call "Read XML Handler.lvclass.vi"("Test Framework in"=w416) -> ("XML Handler.lvclass"=w437:refnum<class "XML Handler.lvclass">, "Test Framework out"=w436:refnum<class "Test Framework.lvclass">)  [unwired: 9 in]
        n169 = call "Finish Temperature.vi"("error in (no error)"=w418, "XML Handler in"=w437) -> ("error out"=w432:errorcluster, "XML Handler out"=w431:refnum<class "XML Handler.lvclass">)  [unwired: 8 in]
        n170 = call "Write Temperature index.vi"("Environmental index"=0 ("Temperature index"), "Test Framework in"=w436) -> ("Test Framework out"=w422:refnum<class "Test Framework.lvclass">)  [unwired: 9 in]
        n171 = call "Close XML.vi"("error in (no error)"=w432, "XML Handler in"=w431) -> ("error out"=w430:errorcluster)  [unwired: 8 in, 1 out]
        n172 = call-poly "Enqueue Message.vi"("Message Data"=Display_states."Start up" ("type"), "Message"=States."Update Display", "Message Queue"=w434) -> ("error out"=w429:errorcluster)  [unwired: 7 in, 1 out]
        n173 = call-dynamic "Read Play sound when done.vi"("Test Framework in"=w422) -> ("Play sound when done"=w420:bool, "Test Framework out"=w421:refnum<class "Test Framework.lvclass">)  [unwired: 9 in]
        n174 = Merge Errors(w429, w430) -> (w428:errorcluster)
        n175 = case shown="True" w420 {
          frame False {
          }
          frame True {
            w444 = T15 0 items=["Finite Samples", "Continuous Samples"] ("sample mode")
            n176 = call-poly <vilib>:"Sound File Info.vi"("path"=path "C:/Windows/Media/notify.wav") -> ("error out"=w438:errorcluster, "sound format"=w443:T16, "total number of samples/ch"=w445:u32, "path out"=w441:path)  [unwired: 7 in]
            n177 = call <vilib>:"Sound File Read Simple.vi"("error in (no error)"=w438, "path"=w441) -> ("error out"=w439:errorcluster, "data"=w453:waveform(dbl)[])  [unwired: 6 in, 2 out]
            n178 = call <vilib>:"Sound Output Configure.vi"("number of samples/ch"=w445, "sample mode"=w444, "error in (no error)"=w439, "sound format"=w443) -> ("error out"=w440:errorcluster, "task ID"=w454:T17)  [unwired: 6 in]
            n179 = call-poly <vilib>:"Sound Output Write.vi"("error in (no error)"=w440, "data"=w453, "task ID"=w454) -> ("error out"=w447:errorcluster, "task ID out"=w448:T17)  [unwired: 7 in]
            n180 = call <vilib>:"Sound Output Start.vi"("error in (no error)"=w447, "task ID"=w448) -> ("error out"=w451:errorcluster, "task ID out"=w452:T17)  [unwired: 8 in]
            n181 = call <vilib>:"Sound Output Wait.vi"("error in (no error)"=w451, "task ID"=w452) -> ("error out"=w449:errorcluster, "task ID out"=w450:T17)  [unwired: 8 in]
            n182 = call <vilib>:"Sound Output Clear.vi"("error in (no error)"=w449, "task ID"=w450) -> ("error out"=w446:errorcluster)  [unwired: 9 in]
            n183 = call <vilib>:"Clear Errors.vi"("error in (no error)"=w446) -> ()  [unwired: 5 in, 2 out]
          }
        }
        n184 = Unbundle By Name(w423) -> ("CtrlWithKeyFocus"=w424:refnum<vi>)
        n185 = Not A Number/Path/Refnum?(number/path/refnum=w424) -> (NaN/Path/Refnum?=w425:bool)
        n186 = case shown="False" w425 {
          tunnel: w424 -> [w455 _]
          frame False {
            n187 = property class="Ctl"(reference=w455, "Key Focus"=TRUE) -> ()  [unwired: 1 in, 2 out]
          }
          frame True {
          }
        }
      }
      frame "Menu Selection" {
        n188 = Variant To Data(error in=w470, type=cluster{string, variant} {"", variant}, Variant=w469) -> (data=w464:cluster{string, variant}, error out=w467:errorcluster)
        n189 = Unbundle(w464) -> (w463:string, w462:variant)
        n190 = case shown="\"Device.info.Load.xml\"" w463 {
          selector: w463 -> [w478 _ _ w510 _ _ _ _ w611]
          tunnel: w467 -> [w479 w492 w502 w512 w563 w586 w590 w597 w614]
          tunnel: [w480 w494 w498 w511 w562 w585 w589 w594 w616] -> w466
          tunnel: w462 -> [_ w490 w501 w508 _ w584 _ _ w613]
          tunnel: w461 -> [w473 w493 w495 w506 w566 w581 w588 w599 w617]
          tunnel: [w473 w493 w495 w506 w566 w587 w588 w598 w617] -> w460
          tunnel: w459 -> [_ _ _ _ w565 _ _ _ _]
          tunnel: w458 -> [_ _ _ _ _ _ _ w596 _]
          tunnel: [_ _ _ _ _ _ _ w593 _] -> w457
          frame "Device.info.Default", "Device.info.Load" {
            n191 = Equal?(x="Device.info.Default", y=w478) -> (x = y?=w476:bool)
            n192 = call "Read Device info parameters Ini file.vi"("Error In"=w479, "Read defaults"=w476) -> ("Error Out"=w480:errorcluster, "Parameter names only"=w475:string[][], "Instrument info"=w474:string[][], "Cancelled"=w472:bool)  [unwired: 6 in]
            n193 = case shown="False" w472 {
              tunnel: w476 -> [w484 _]
              tunnel: w475 -> [w483 _]
              tunnel: w474 -> [w482 _]
              frame False {
                n194 = Select(t=w483, s=w484, f=w482) -> (s? t:f=w481:string[][])
                n195 = local write "Device Information"(w481) -> ()
              }
              frame True {
              }
            }
          }
          frame "Device.info.Save" {
            n196 = Variant To Data(error in=w492, type=path "" ("base path"), Variant=w490) -> (data=w488:path, error out=w491:errorcluster)
            n197 = Build Path(base path=w488, name or relative path="Device info") -> (appended path=w485:path)
            n198 = local read "Device Information"() -> (w486:string[][])
            n199 = call "Write Device info parameters Ini file.vi"("Instrument info"=w486, "Error In"=w491, "Start path"=w485) -> ("Error Out"=w494:errorcluster)  [unwired: 8 in]
          }
          frame "Device.info.Load.xml" {
            n200 = Variant To Data(error in=w502, type=path "", Variant=w501) -> (data=w499:path, error out=w498:errorcluster)
            n201 = call "Read Device Information from XML.vi"("XML File Path"=w499) -> ("Canceled"=w496:bool, "info out"=w497:string[][])  [unwired: 9 in]
            n202 = case shown="True" w496 {
              tunnel: w497 -> [w503 _]
              frame False {
                n203 = local write "Device Information"(w503) -> ()
              }
              frame True {
              }
            }
          }
          frame Default {
            # "Execute independent vi's."
            n204 = case shown="\"de-embed\"" w510 {
              tunnel: [_ "DUT+Fixture (folder)" ("Control Name") "SnP File Path" ("Control Name") "File Path" ("Control Name") "" ("Control Name") _ _ _ _] -> w509
              tunnel: [_ w551 w552 w555 w557 w558 w559 w560 w561] -> w505
              frame Default {
              }
              frame "de-embed" {
                n205 = vi-ref "De-embed S-parameters.vi"() -> (w551:refnum<vi>)
              }
              frame "Parameter Extractor" {
                n206 = vi-ref "Extraction - MainUI.vi"() -> (w552:refnum<vi>)
              }
              frame "Switching Time Extractor" {
                n207 = vi-ref "MainUI.vi"() -> (w555:refnum<vi>)
              }
              frame "Program OTP" {
                n208 = vi-ref "OTP - Main UI.vi"() -> (w557:refnum<vi>)
              }
              frame "Acquire Oscilloscope trace" {
                n209 = vi-ref "Fetch Oscilloscope trace.vi"() -> (w558:refnum<vi>)
              }
              frame "WS1021 GUI" {
                n210 = vi-ref "WS1021.lvclass:WS1021 GUI.vi"() -> (w559:refnum<vi>)
              }
              frame "Read OS info" {
                n211 = vi-ref "Read OS.vi"() -> (w560:refnum<vi>)
              }
              frame "ISD batch file generator" {
                n212 = vi-ref "Make ISD batch file.vi"() -> (w561:refnum<vi>)
              }
            }
            n213 = Not A Number/Path/Refnum?(number/path/refnum=w505) -> (NaN/Path/Refnum?=w504:bool)
            n214 = Empty String/Path?(string/path=w509) -> (empty?=w507:bool)
            n215 = case shown="False" w504 {
              tunnel: w512 -> [w529 w549]
              tunnel: [w528 w549] -> w511
              tunnel: w508 -> [w516 _]
              tunnel: w509 -> [w515 _]
              tunnel: w507 -> [w514 _]
              tunnel: w505 -> [w513 _]
              frame False {
                n216 = invoke class="VI" method="FP.Open"(reference=w513, error in=w529, "Activate"=TRUE ("Activate?"), "State"=T8."Standard") -> (reference out=w521:refnum<vi>, error out=w525:errorcluster)  [unwired: 1 in, 3 out]
                n217 = property class="VI" props=["Exec.State", "IsSmartProbe"](reference=w521, error in=w525) -> (reference out=w523:refnum<vi>, error out=w524:errorcluster, "Exec.State"=w522:T18)  [unwired: 1 out]
                n218 = case shown="\"Run top level\"" w522 {
                  tunnel: [w539 w544 w546 w548] -> w520
                  tunnel: w524 -> [w539 w542 w546 w548]
                  tunnel: w523 -> [w538 w541 w545 w547]
                  tunnel: [w538 w540 w545 w547] -> w519
                  frame "Bad", Default {
                  }
                  frame "Idle" {
                    n219 = invoke class="VI" method="Run VI"(reference=w541, error in=w542, "Wait until done"=FALSE ("Wait Until Done")) -> (reference out=w540:refnum<vi>, error out=w544:errorcluster)  [unwired: 2 in, 3 out]
                  }
                  frame "Run top level" {
                  }
                  frame "Running" {
                  }
                }
                n220 = case shown="False" w514 {
                  tunnel: w520 -> [w535 w537]
                  tunnel: w519 -> [w534 w536]
                  tunnel: [w533 w536] -> w518
                  tunnel: [w532 w537] -> w517
                  tunnel: w516 -> [w531 _]
                  tunnel: w515 -> [w530 _]
                  frame False {
                    n221 = invoke class="VI" method="Ctrl Val.Set"(reference=w534, error in=w535, "Control Name"=w530, "Value"=w531) -> (reference out=w533:refnum<vi>, error out=w532:errorcluster)  [unwired: 1 in, 3 out]
                  }
                  frame True {
                  }
                }
                n222 = Close Reference(reference=w518, error in (no error)=w517) -> (error out=w528:errorcluster)
              }
              frame True {
              }
            }
          }
          frame "About" {
            n223 = case shown="True" w565 {
              tunnel: [w569 w572] -> w564
              tunnel: w563 -> [w567 w580]
              tunnel: [w568 w574] -> w562
              frame False {
                n224 = Get Date/Time String() -> (date string=w571:string)  [unwired: 3 in, 1 out]
                n225 = Format Into String(format string="WiSpry Test Framework\nSource Code version %s" ("message"), error in=w567, w571) -> (resulting string=w569:string, error out=w568:errorcluster)  [unwired: 1 in]
              }
              frame True {
                n226 = Current VI's Path() -> (path=w579:path)
                n227 = Strip Path(path=w579) -> (stripped path=w578:path)  [unwired: 1 out]
                n228 = Strip Path(path=w578) -> (stripped path=w577:path)  [unwired: 1 out]
                n229 = call <vilib>:"FileVersionInfo.vi"("error in (no error)"=w580, "Application Path in"=w577) -> ("error out"=w575:errorcluster, "File Version Info"=w573:string)  [unwired: 6 in, 2 out]
                n230 = Format Into String(format string="WiSpry Test Framework\nExecutable version %s" ("message"), error in=w575, w573) -> (resulting string=w572:string, error out=w574:errorcluster)  [unwired: 1 in]
              }
            }
            n231 = One Button Dialog(message=w564) -> ()  [unwired: 1 in, 1 out]
          }
          frame "Sound" {
            n232 = Variant To Data(error in=w586, type=FALSE, Variant=w584) -> (data=w582:bool, error out=w585:errorcluster)
            n233 = call-dynamic "Write Play sound when done.vi"("Play sound when done"=w582, "Test Framework in"=w581) -> ("Test Framework out"=w587:refnum<class "Test Framework.lvclass">)  [unwired: 9 in]
          }
          frame "Save Setup" {
            n234 = Flatten To XML(6:w588) -> (2:w591:string)
            n235 = call-poly <vilib>:"Write to XML File.vi"("error in (no error)"=w590, "XML Input"=w591) -> ("error out"=w589:errorcluster)  [unwired: 7 in, 2 out]
          }
          frame "Load Setup" {
            n236 = call "Load user settings.vi"("error in (no error)"=w597, "Test Framework in"=w599) -> ("error out"=w595:errorcluster, "Canceled"=w592:bool, "Test Framework out"=w598:refnum<class "Test Framework.lvclass">)  [unwired: 7 in]
            n237 = case shown="False" w592 {
              tunnel: w596 -> [w603 _]
              tunnel: w595 -> [w602 w605]
              tunnel: [w601 w605] -> w594
              tunnel: [w600 FALSE ("event data")] -> w593
              frame False {
                w600 = TRUE ("event data")
                n238 = Generate User Event(user event=w603, event data cluster=w600, error in=w602) -> (error out=w601:errorcluster)  [unwired: 1 in, 1 out]
              }
              frame True {
              }
            }
          }
          frame "guide.OTPcal", "guide.UG" {
            n239 = Variant To Data(error in=w614, type=path "", Variant=w613) -> (error out=w615:errorcluster)  [unwired: 1 out]
            n240 = Current VI's Path() -> (path=w608:path)
            n241 = case shown="\"guide.UG\"" w611 {
              tunnel: [_ "Help files\\WiSpry Test Framework - OTP calibration.pdf" "Help files\\WiSpry Test Framework - User Guide.pdf"] -> w610
              frame "False", Default {
              }
              frame "guide.OTPcal" {
              }
              frame "guide.UG" {
              }
            }
            n242 = Strip Path(path=w608) -> (stripped path=w607:path)  [unwired: 1 out]
            n243 = Strip Path(path=w607) -> (stripped path=w606:path)  [unwired: 1 out]
            n244 = Build Path(base path=w606, name or relative path=w610) -> (appended path=w609:path)
            n245 = call <vilib>:"Open a Document on Disk.vi"("error in (no error)"=w615, "document path"=w609) -> ("error out"=w616:errorcluster)  [unwired: 5 in]
          }
        }
      }
    }
    n246 = call "Error Handler - Message Handling Loop.vi"("error in (no error)"=w29, "Message Queue"=w28) -> ("dup error in"=w27:errorcluster)  [unwired: 8 in, 1 out]
  }
  "Test Framework.lvclass Out" <- w17
  n247 = while {
    tunnel: w16 -> [w629]
    shift-right: [w625] -> w13
    shift-left: w15 -> [w628]
    tunnel: [w623] -> w14
    shift-right: [w621] -> _
    shift-left: _ -> [w620]
    stop <- w624 stop-if-true
    # "Evten Handling Loop"
    n248 = event shown="[8] \"Run Measurements Button\": Value Change" {
      selector: w628 -> [_ _ _ _ _ _ _ _ _ _ _ _ _ _ _]
      dyn-events: [_ _ _ _ _ _ _ _ _ _ _ _ _ _ _] -> w625
      timeout: 250 -> [_ _ _ _ _ _ _ _ _ _ _ _ _ _ _]
      tunnel: w629 -> [w633 w647 w655 w666 w699 w703 w707 w712 w721 w731 w742 w752 w754 w762 w775]
      tunnel: [w631 _ w657 w668 w697 w701 w705 w710 w726 w733 w740 _ _ w759 _] -> w627
      tunnel: [w630 w647 w656 w667 w698 w702 w706 w711 w727 w732 w741 w752 w754 w761 w775] -> w626
      tunnel: [_ _ _ _ _ _ _ _ _ _ _ _ _ _ TRUE] -> w624
      tunnel: [_ w635 _ w664 _ _ _ _ w723 _ _ _ _ _ _] -> w621
      tunnel: w620 -> [_ _ _ w664 _ _ _ _ w723 _ _ _ _ _ _]
      event Panel Close? {
        n249 = event-data() -> ()  [unwired: 1 in, 1 out]
        n250 = call-poly "Enqueue Message.vi"("Message"=States."Exit", "Message Queue"=w633) -> ("error out"=w631:errorcluster, "dup Message Queue"=w630:refnum<queue>)  [unwired: 8 in]
        n251 = event-data("Discard?"=TRUE) -> ()  [unwired: 1 in, 1 out]
      }
      event Timeout {
        n252 = event-data() -> ()  [unwired: 1 in, 1 out]
        n253 = Get Date/Time String(want seconds? (F)=TRUE) -> (date string=w645:string, time string=w646:string)  [unwired: 2 in]
        n254 = Concatenate Strings(w645, "\n" ("string"), w646) -> (→"Time String":string)
        n255 = control-ref of="This VI"() -> (w639:refnum<vi>)
        n256 = control-ref of="String"() -> (w638:refnum<vi>)
        n257 = invoke class="VI" method="FindCtrlWithKeyFocus"(reference=w639) -> ("FindCtrlWithKeyFocus"=w641:refnum<vi>, "CtrlFound?"=w640:bool)  [unwired: 3 in, 2 out]
        n258 = property class="Str"(reference=w638) -> (reference out=w636:refnum<vi>, "Key Focus"=w637:bool)  [unwired: 1 in, 1 out]
        n259 = case shown="False" w640 {
          tunnel: w641 -> [_ w652]
          tunnel: [w649 w652] -> w635
          tunnel: w637 -> [w651 _]
          tunnel: w636 -> [w650 _]
          frame False {
            n260 = Select(t=w650, s=w651, f=refnum<k0> refnum) -> (s? t:f=w649:refnum<vi>)
          }
          frame True {
          }
        }
      }
      event "Exit Button": Value Change {
        n261 = event-data() -> ()  [unwired: 1 in, 4 out]
        n262 = call-poly "Enqueue Message.vi"("Priority Message? (F)"=TRUE, "Message"=States."Exit", "Message Queue"=w655) -> ("error out"=w657:errorcluster, "dup Message Queue"=w656:refnum<queue>)  [unwired: 7 in]
      }
      event "Test Listbox": Mouse Down {
        n263 = event-data() -> ("CtlRef"=w665:refnum<vi>, "Coords"=w660:T19, "Button"=w663:u16, "Mods"=w658:cluster{"Double Click":bool, "Menu Key":bool})  [unwired: 1 in, 1 out]
        n264 = Unbundle(w660) -> ("Horizontal"=w662:i32)  [unwired: 1 out]
        n265 = Less?(x=w662, y=56) -> (x < y?=w659:bool)
        n266 = case shown="False" w659 {
          tunnel: w663 -> [_ _]
          tunnel: [w672 w688] -> w668
          tunnel: [w673 w687] -> w667
          tunnel: w666 -> [w671 w686]
          tunnel: w665 -> [_ w683]
          tunnel: w658 -> [w670 _]
          frame False {
            n267 = Unbundle(w670) -> ("Double Click"=w669:bool)  [unwired: 1 out]
            n268 = case shown="True" w669 {
              tunnel: [w674 w678] -> w673
              tunnel: [_ w677] -> w672
              tunnel: w671 -> [w674 w676]
              frame False {
              }
              frame True {
                n269 = property on="Test Listbox" class="LstBox (strict)"() -> ("Item Names"=w681:string[], "Value"=w675:i32)  [unwired: 2 in, 2 out]
                n270 = Index Array(array=w681, index=w675) -> (element=w680:string)
                n271 = call-poly "Enqueue Message.vi"("Message Data"=w680, "Message"=States."Configure Test", "Message Queue"=w676) -> ("error out"=w677:errorcluster, "dup Message Queue"=w678:refnum<queue>)  [unwired: 7 in]
              }
            }
          }
          frame True {
            w689 = 37
            n272 = property class="LstBox (strict)"(reference=w683) -> (reference out=w692:refnum<vi>, "Item Symbols"=w693:i32[], "Value"=w682:i32)  [unwired: 1 in, 1 out]
            n273 = Index Array(array=w693, index=w682) -> (element=w690:i32)
            n274 = Equal?(x=w690, y=w689) -> (x = y?=w691:bool)
            n275 = Select(t=38, s=w691, f=w689) -> (s? t:f=w694:i32)
            n276 = Replace Array Subset(array=w693, new element=w694, index=w682) -> (w684:i32[])
            n277 = property class="LstBox (strict)"(reference=w692, "Item Symbols"=w684) -> ()  [unwired: 1 in, 2 out]
            n278 = call-poly "Enqueue Message.vi"("Message Data"=w684, "Message"=States."Update test list", "Message Queue"=w686) -> ("error out"=w688:errorcluster, "dup Message Queue"=w687:refnum<queue>)  [unwired: 7 in]
          }
        }
      }
      event "Assign Instr Button": Value Change {
        n279 = event-data() -> ()  [unwired: 1 in, 1 out]
        n280 = call-poly "Enqueue Message.vi"("Message"=States."Assign Instruments", "Message Queue"=w699) -> ("error out"=w697:errorcluster, "dup Message Queue"=w698:refnum<queue>)  [unwired: 8 in]
      }
      event "Conf temp and DC Button": Value Change {
        n281 = event-data() -> ()  [unwired: 1 in, 1 out]
        n282 = call-poly "Enqueue Message.vi"("Message"=States."Configure Evironmental", "Message Queue"=w703) -> ("error out"=w701:errorcluster, "dup Message Queue"=w702:refnum<queue>)  [unwired: 8 in]
      }
      event "Conf Device Button": Value Change {
        n283 = event-data() -> ()  [unwired: 1 in, 1 out]
        n284 = call-poly "Enqueue Message.vi"("Message"=States."Configure Device", "Message Queue"=w707) -> ("error out"=w705:errorcluster, "dup Message Queue"=w706:refnum<queue>)  [unwired: 8 in]
      }
      event "Configure Measurements Button": Value Change {
        n285 = event-data() -> ()  [unwired: 1 in, 1 out]
        n286 = property on="Test Listbox" class="LstBox (strict)"() -> ("Item Names"=w714:string[])  [unwired: 2 in, 2 out]
        n287 = Index Array(array=w714, index="Test Listbox") -> (element=w708:string)
        n288 = call-poly "Enqueue Message.vi"("Message Data"=w708, "Message"=States."Configure Test", "Message Queue"=w712) -> ("error out"=w710:errorcluster, "dup Message Queue"=w711:refnum<queue>)  [unwired: 7 in]
      }
      event "Run Measurements Button": Value Change {
        # "Run:\n- Change data path\n- Update device info\n- Init XML\n- Update Display\n- Init Environmental\n- Next Environmental\n- Run Tests OR Finish test"
        n289 = event-data() -> ()  [unwired: 1 in, 1 out]
        n290 = property on="Data Path" class="Path"() -> ("Value"=w716:path)  [unwired: 2 in, 2 out]
        n291 = property on="File Name" class="Str"() -> ("Value"=w717:string)  [unwired: 2 in, 2 out]
        n292 = Build Path(base path=w716, name or relative path=w717) -> (appended path=w718:path)
        n293 = Bundle("appended path"=w718, "appended path"=w718) -> (w715:T20)  [unwired: 1 in]
        n294 = call-poly "Enqueue Message.vi"("Message Data"=w715, "Message"=States."Change Data Path", "Message Queue"=w721) -> ("error out"=w722:errorcluster, "dup Message Queue"=w720:refnum<queue>)  [unwired: 7 in]
        n295 = call-poly "Enqueue Message.vi"("error in (no error)"=w722, "Message Data"=w723, "Message"=States."Update device info", "Message Queue"=w720) -> ("error out"=w728:errorcluster, "dup Message Queue"=w729:refnum<queue>)  [unwired: 6 in]
        n296 = call-poly "Enqueue Message.vi"("error in (no error)"=w728, "Message"=States."Init XML", "Message Queue"=w729) -> ("error out"=w726:errorcluster, "dup Message Queue"=w727:refnum<queue>)  [unwired: 7 in]
      }
      event "Calibrate Paths Button": Value Change {
        n297 = event-data() -> ()  [unwired: 1 in, 3 out]
        n298 = call-poly "Enqueue Message.vi"("Message"=States."Calibrate Path", "Message Queue"=w731) -> ("error out"=w733:errorcluster, "dup Message Queue"=w732:refnum<queue>)  [unwired: 8 in]
      }
      event "Data Path": Value Change {
        n299 = event-data() -> ("OldVal"=w736:path)  [unwired: 1 in]
        n300 = Build Path(base path="Data Path", name or relative path="File Name") -> (appended path=w735:path)
        n301 = Bundle("appended path"=w735, "OldVal"=w736) -> (w734:cluster{"appended path":path, "OldVal":path})  [unwired: 1 in]
        n302 = call-poly "Enqueue Message.vi"("Message Data"=w734, "Message"=States."Change Data Path", "Message Queue"=w742) -> ("error out"=w740:errorcluster, "dup Message Queue"=w741:refnum<queue>)  [unwired: 7 in]
      }
      event "OpenFolder": Value Change {
        n303 = event-data() -> ()  [unwired: 1 in, 1 out]
        n304 = local read "Data Path"() -> (w750:path)
        n305 = List Folder(path=w750) -> (path out=w745:path, filenames=w747:string[], error out=w748:errorcluster)  [unwired: 3 in, 1 out]
        n306 = Index Array(array=w747) -> (element=w749:string)  [unwired: 1 in]
        n307 = Build Path(base path=w745, name or relative path=w749) -> (appended path=w744:path)
        n308 = Empty Array?(array=w747) -> (empty?=w746:bool)
        n309 = Select(t=w745, s=w746, f=w744) -> (s? t:f=w743:path)
        n310 = call <vilib>:"Show in File System.vi"("error in (no error)"=w748, "file or directory path"=w743) -> ("error out"=w751:errorcluster)  [unwired: 9 in]
        n311 = case shown="No Error" w751 {
          frame No Error {
          }
          frame Error {
            n312 = One Button Dialog(message="Folder not found") -> ()  [unwired: 1 in, 1 out]
          }
        }
      }
      event Menu Selection (App) {
        n313 = event-data() -> ()  [unwired: 1 in, 1 out]
      }
      event Menu Selection (User) {
        n314 = event-data() -> ("ItemTag"=w756:string, "MenuRef"=w755:refnum<k9>)  [unwired: 1 in]
        n315 = case shown="Default" w756 {
          selector: w756 -> [w763 w767]
          tunnel: cluster{string, variant} {"", variant} -> [w766 w773]
          tunnel: [w765 w772] -> w757
          tunnel: w755 -> [_ w771]
          frame Default {
            n316 = local read "Data Path"() -> (w764:path)
            n317 = Bundle(cluster=w766, w763, w764) -> (w765:cluster{string, variant})
          }
          frame "Sound" {
            n318 = Get Menu Item Info(7:w767, 11:w771) -> (3:w770:refnum<k9>, 4:w769:bool)  [unwired: 1 in, 5 out]
            n319 = Not(x=w769) -> (.not. x?=w768:bool)
            n320 = Set Menu Item Info(6:w768, 7:w767, 11:w770) -> ()  [unwired: 4 in, 2 out]
            n321 = Bundle(cluster=w773, w767, w768) -> (w772:cluster{string, variant})
          }
        }
        n322 = call-poly "Enqueue Message.vi"("Message Data"=w757, "Message"=States."Menu Selection", "Message Queue"=w762) -> ("error out"=w759:errorcluster, "dup Message Queue"=w761:refnum<queue>)  [unwired: 7 in]
      }
      event User Event {
        n323 = event-data() -> ()  [unwired: 1 in, 4 out]
      }
    }
    n324 = call "Error Handler - Event Handling Loop.vi"("error in (no error)"=w627, "Message Queue"=w626) -> ("dup error in"=w623:errorcluster)  [unwired: 8 in, 1 out]
  }
  n325 = Unregister For Events(event registration refnum=w13, error in=w14) -> (error out=w12:errorcluster)
  n326 = Close File(refnum=w4) -> ()  [unwired: 1 in, 2 out]
  n327 = Merge Errors(w12, w11) -> (w9:errorcluster)
  n328 = call "Destroy User Event - Stop.vi"("error in (no error)"=w9, "User Event - Stop"=w10) -> ("error out"=w7:errorcluster)  [unwired: 9 in]
  n329 = disable-structure shown="Enabled" {
    disable-tunnel: w7 -> [w777 w778]
    disable-tunnel: [w776 w778] -> w6
    frame Disabled {
      n330 = invoke class="VI" method="FP.Close"(error in=w777) -> (error out=w776:errorcluster)  [unwired: 2 in, 2 out]
    }
    frame Enabled {
    }
  }
  "Error Out" <- w6
